vi "project1.vi"() -> ()   [LabVIEW 2014]
uses:
  <vilib>/ptbypt/Frequency Domain.llb/Real FFT PtByPt.vi
  <vilib>/Analysis/3filter.llb/Chebyshev Filter (CDB).vi
  <vilib>/ptbypt/NI_PtbyPt.lvlib
  <vilib>/Analysis/NI_AALBase.lvlib
panel:
  in  "Tab Control":enum32{"SINE", "FOURIER SINE"}(tab)
  in  "Amplitude 2":dbl(knob) scale=0.0..100.0
  in  "Frequency 2":dbl(knob) scale=0.0..100.0
  in  "Amplitude 1":dbl(knob) scale=0.0..100.0
  in  "Frequency 1":dbl(knob) scale=0.0..100.0
  in  "stop 2":bool
  out "Sine":dynamicdata(graph)
  out "Waveform Graph":dbl[](graph)
  in  "stop":bool
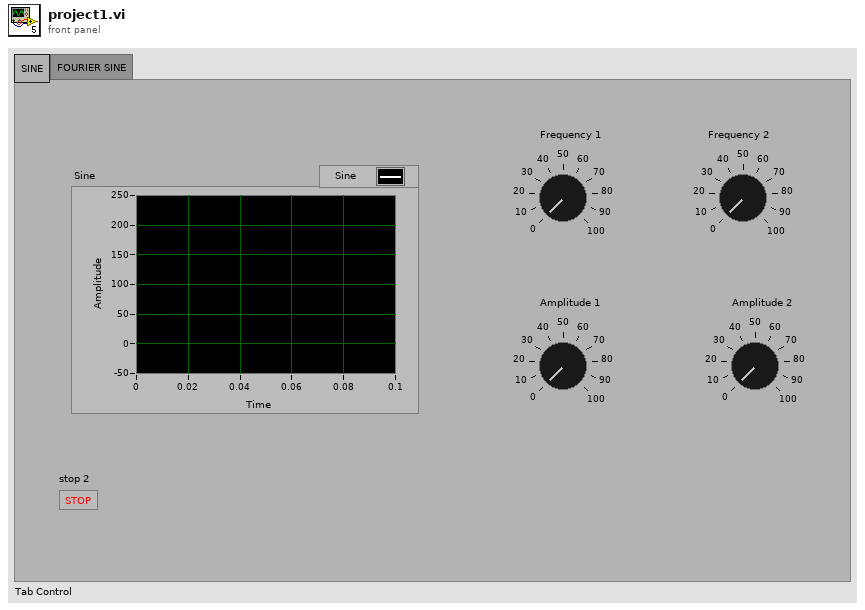
[diagram p1: front panel]
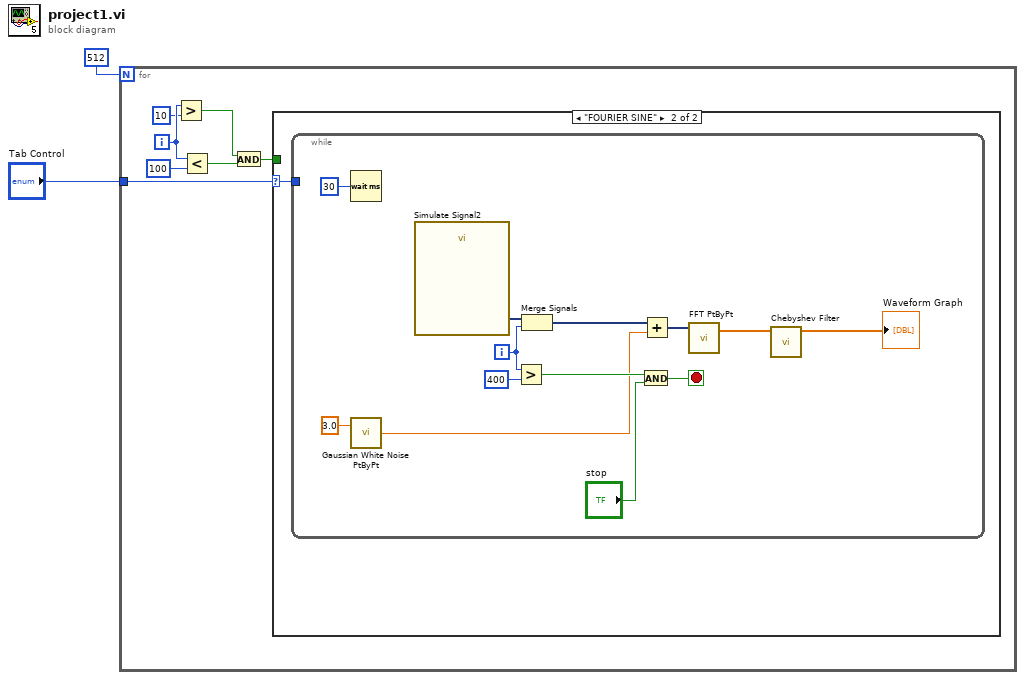
[diagram p0: block diagram]
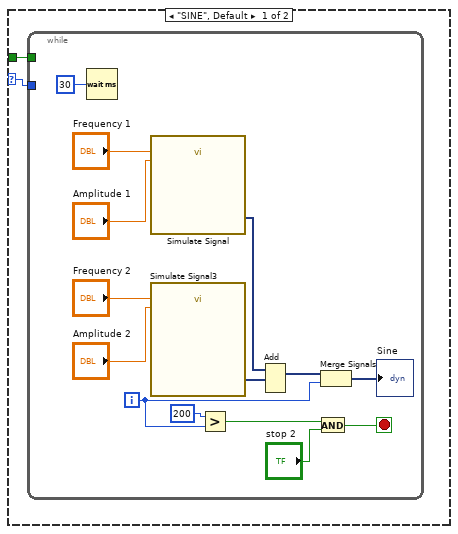
[diagram p2: hidden frame]
diagram:
  n1 = for {
    N: 512 -> [_]
    tunnel: "Tab Control" -> [w9]
    i -> [w8]
    n2 = Greater?(x=w8, y=10) -> (0:w5:bool)
    n3 = Less?(x=w8, y=100) -> (x < y?=w4:bool)
    n4 = And(x=w5, y=w4) -> (x .and. y?=w3:bool)
    n5 = case shown="\"FOURIER SINE\"" w9 {
      selector: w9 -> [w10 w26]
      tunnel: w3 -> [w11 _]
      frame "SINE", Default {
        n6 = while {
          tunnel: w11 -> [_]
          tunnel: w10 -> [_]
          i -> [w20]
          stop <- w22 stop-if-true
          n7 = Wait (ms)(milliseconds to wait=u32 30) -> ()  [unwired: 1 out]
          n8 = call "Simulate Signal"("Frequency"="Frequency 1", "Amplitude"="Amplitude 1") -> ("Sine"=w17:dynamicdata)  [unwired: 12 in, 1 out]
          n9 = call "Simulate Signal3"("Frequency"="Frequency 2", "Amplitude"="Amplitude 2") -> ("Sine"=w16:dynamicdata)  [unwired: 12 in, 1 out]
          n10 = Greater?(x=200, y=w20) -> (0:w24:bool)
          n11 = Add(1:w16, 2:w17) -> (0:w18:dynamicdata)  [unwired: 1 in, 1 out]
          n12 = And(x=w24, y="stop 2") -> (x .and. y?=w22:bool)
          n13 = Merge Signals(w18, w20) -> (→"Sine":dynamicdata)
        }
      }
      frame "FOURIER SINE" {
        n14 = while {
          tunnel: w26 -> [_]
          i -> [w33]
          stop <- w36 stop-if-true
          n15 = Wait (ms)(milliseconds to wait=u32 30 ("millisecond timer value")) -> ()  [unwired: 1 out]
          n16 = call <vilib>:"Gaussian White Noise PtByPt.vi"("standard deviation"=3.0) -> ("Gaussian white noise"=w31:dbl)  [unwired: 2 in]
          n17 = call "Simulate Signal2"() -> ("Sine"=w34:dynamicdata)  [unwired: 14 in, 1 out]
          n18 = Greater?(x=w33, y=400) -> (0:w38:bool)
          n19 = Merge Signals "Merge Signals"(w34, w33) -> (w32:dynamicdata)
          n20 = And(x=w38, y="stop") -> (x .and. y?=w36:bool)
          n21 = Add(x=w32, y=w31) -> (x+y=w29:dynamicdata)
          n22 = call-poly <vilib>:"FFT PtByPt.vi"("x"=w29) -> ("FFT{X}"=w28:cdb[])  [unwired: 3 in, 1 out]
          n23 = call-poly <vilib>:"Chebyshev Filter.vi"("X"=w28) -> ("Filtered X"=→"Waveform Graph":cdb[])  [unwired: 9 in, 1 out]
        }
      }
    }
  }
